vi "Get Exit Code.vi"(8 "error in":errorcluster, 10 "ignore error if still active (T)":bool=TRUE, 11 "pipe in":T1) -> (0 "error out":errorcluster, 1 "exited?":bool, 2 "exit code":i32, 3 "pipe out":T1, 5 "running?":bool)   [LabVIEW 2013, in "LV Process library.lvlib"]
doc: "Calls lv_proc.dll and reads process exit code. Error is returned if process has not exited yet and 259 value (STILL_ACTIVE) is returned as an exit code. Optionally STILL_ACTIVE error can be filtered by 'ignore error if still active' (default)."
uses:
  LV Process library.lvlib
  Pipe Handle.ctl
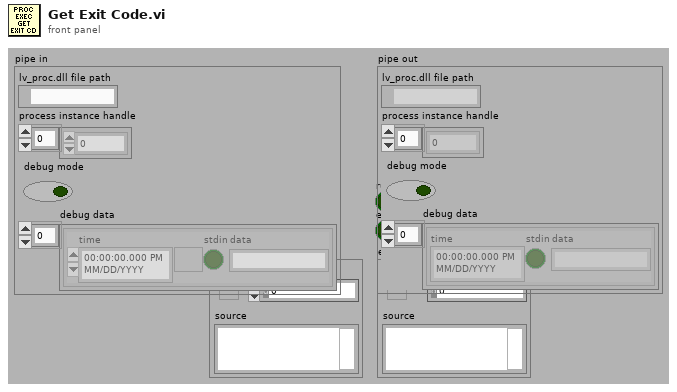
[diagram p1: front panel]
types:
  T1 = typedef "LV Process library.lvlib/Pipe Handle.ctl" = cluster{"lv_proc.dll file path":path, "process instance handle":u32[], "debug mode":bool, "debug data":cluster{"time":timestamp, "stdin":bool, "data":string}[]}
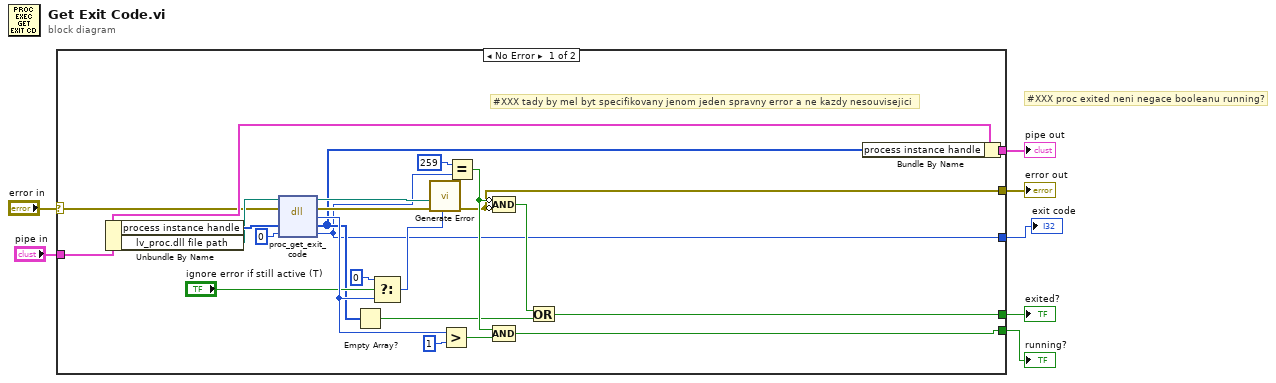
[diagram p0: block diagram]
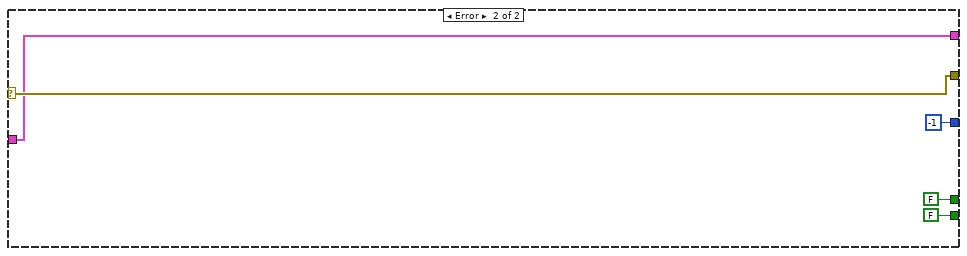
[diagram p2: hidden frame]
diagram:
  # "#XXX proc exited neni negace booleanu running?"
  n1 = case shown="No Error" "error in" {
    selector: "error in" -> [w12 w35]
    tunnel: "pipe in" -> [w23 w34]
    tunnel: [w16 w35] -> w6
    tunnel: [w11 w34] -> w4
    tunnel: [w10 FALSE] -> w3
    tunnel: [w9 FALSE] -> w2
    tunnel: [w8 -1 ("code")] -> w1
    frame No Error {
      # "#XXX tady by mel byt specifikovany jenom jeden spravny error a ne kazdy nesouvisejici"
      n2 = Unbundle By Name(w23) -> ("process instance handle"=w25:u32[], "lv_proc.dll file path"=w24:path)
      n3 = dll-call lib="lv_proc.dll" fn="proc_get_exit_code"(path in=w24, error in=w12, "proc"=w25, "code"=0 ("code mem")) -> (path out=w17:path, error out=w18:errorcluster, "error"=w22:i32, "proc"=w15:u32[], "code"=w8:i32)  [unwired: 1 in]
      n4 = Empty Array?(array=w15) -> (empty?=w13:bool)
      n5 = Select(t=0, s="ignore error if still active (T)", f=w22) -> (s? t:f=w19:i32)
      n6 = call "Generate Error.vi"("error code in"=w19, "error in"=w18, "lv_proc.dll path in"=w17) -> ("error out"=w16:errorcluster)  [unwired: 6 in, 1 out]
      n7 = Greater?(x=w22, y=1 ("x")) -> (0:w28:bool)
      n8 = Equal?(x=259, y=w8) -> (x = y?=w26:bool)
      n9 = Compound Arithmetic op=AND(invert w26, invert w16) -> (w14:bool)
      n10 = Compound Arithmetic op=AND(w26, w28) -> (w10:bool)
      n11 = Or(x=w14, y=w13) -> (x .or. y?=w9:bool)
      n12 = Bundle By Name(cluster=w23, "process instance handle"=w15) -> (w11:T1)
    }
    frame Error {
    }
  }
  "error out" <- w6
  "pipe out" <- w4
  "running?" <- w3
  "exited?" <- w2
  "exit code" <- w1
